vi "Sequence.Compile.vi"(8 "error in (no error)":errorcluster, 11 "State Variables":T10={"Aliases.All"=[], "Aliases.Outputs"=[], "UI.Sequence#ofColumns"=0, "SysDef.Path"=path "", "UI.SequenceRef"=refnum, "UI.StepInformationRef"=refnum, "UI.AbortRef"=refnum, "UI.GraphRef"=refnum, "UI.ViewRef"=refnum, "UI.IterationsRef"=refnum, "UI.IterationInformationRef"=refnum, "INI.Settings"={"Build Location"=path "C:/Simple Sequence Editor/SequenceRepo", "LoggingLocation"=path ""}, "NIVS.Workspace Event"=refnum, "UI.SkipChannel"=refnum, "NIVS.Launched?"=FALSE, "UI.DurationChannel"=refnum}) -> (0 "error out":errorcluster, 1 "Warnings":string[](array[string]), 2 "CompiledSettings":T1)   [LabVIEW 2013, in "Simple Sequence Tools - Editor.lvlib"]
uses:
  Simple Sequence Tools - Editor.lvlib
  Types/Main.StateVariables.ctl
  Shared/Types/Channel.Properties.ctl
  Shared/Types/INI.Settings
  Types/Compiled.RTSequenceProperties.ctl
  Types/Compiled.StepProperties.ctl
  Types/Compiled.IOStateProperties.ctl
  Types/Compiled.StepElementProperties.ctl
  Shared/Types/Step.Types.ctl
  Types/Compiled.StepCondition.ctl
  Types/Conditions.OperationTypes.ctl
  Types/Compiled.SequenceChannels.ctl
  Shared/Simple Sequence Tools - Shared.lvlib
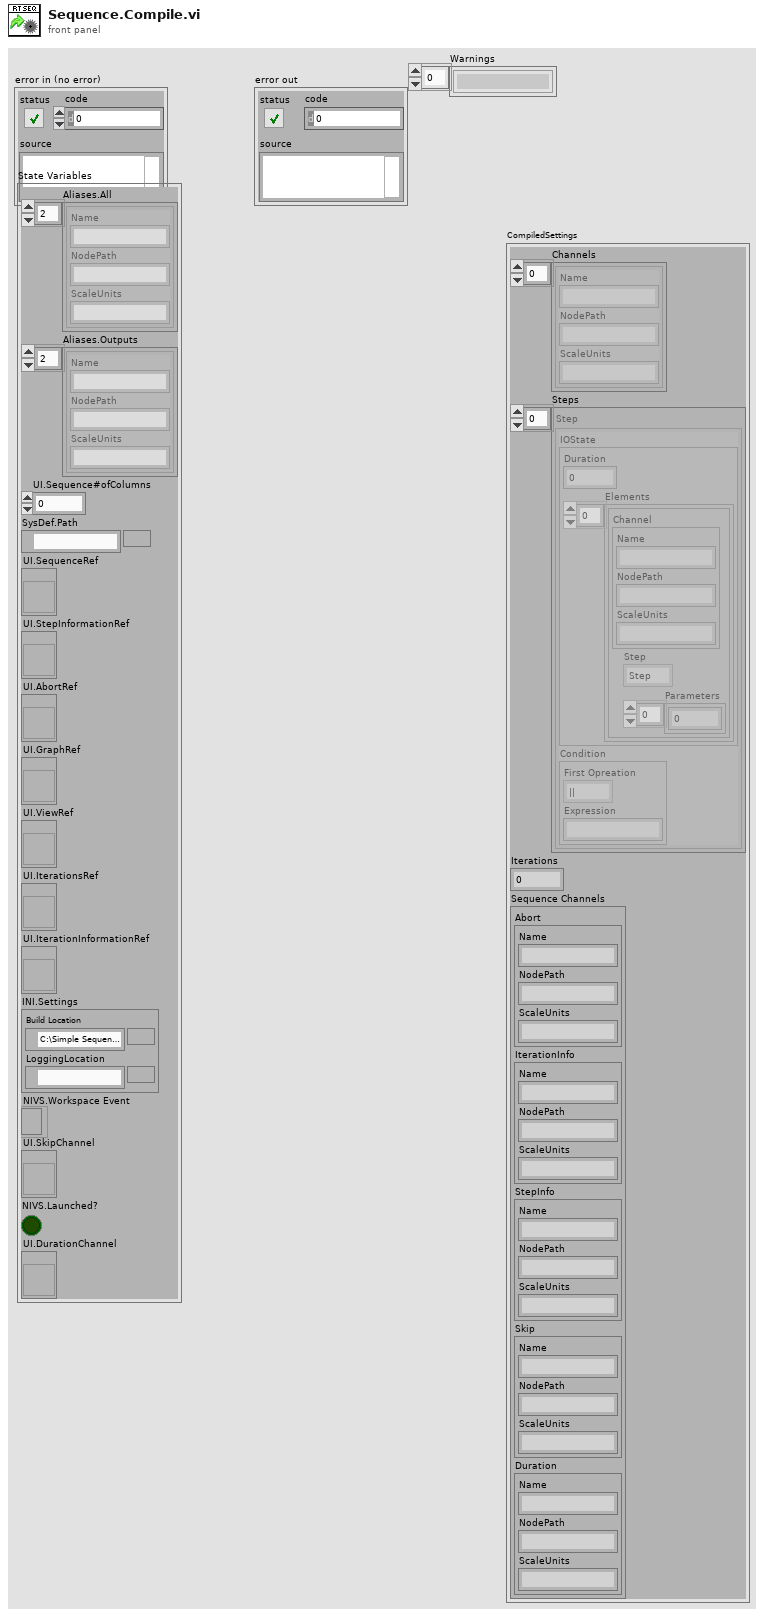
[diagram p1: front panel]
types:
  T1 = typedef "Simple Sequence Tools - Editor.lvlib/Compiled.RTSequenceProperties.ctl" = cluster{"Channels":T2[], "Steps":T3[], "Iterations":u32, "Sequence Channels":T9}
  T2 = typedef "Simple Sequence Tools - Shared.lvlib/Channel.Properties.ctl" = cluster{"Name":string, "NodePath":string, "ScaleUnits":string}
  T3 = typedef "Simple Sequence Tools - Editor.lvlib/Compiled.StepProperties.ctl" = cluster{"IOState":T4, "Condition":T7}
  T4 = typedef "Simple Sequence Tools - Editor.lvlib/Compiled.IOStateProperties.ctl" = cluster{"Duration":dbl, "Elements":T5[]}
  T5 = typedef "Simple Sequence Tools - Editor.lvlib/Compiled.StepElementProperties.ctl" = cluster{"Channel":T2, "Step":T6, "Parameters":dbl[]}
  T6 = typedef "Simple Sequence Tools - Shared.lvlib/Step.Types.ctl" = enum8{"Step", "iStep", "Ramp", "Unchanged", "Unknown", "Sine", "LogSine", "LinearSine", "ForcedRamp"}
  T7 = typedef "Simple Sequence Tools - Editor.lvlib/Compiled.StepCondition.ctl" = cluster{"First Opreation":T8, "Expression":string}
  T8 = typedef "Simple Sequence Tools - Editor.lvlib/Conditions.OperationTypes.ctl" = enum8{"None", "&&", "||"}
  T9 = typedef "Simple Sequence Tools - Editor.lvlib/Compiled.SequenceChannels.ctl" = cluster{"Abort":T2, "IterationInfo":T2, "StepInfo":T2, "Skip":T2, "Duration":T2}
  T10 = typedef "Simple Sequence Tools - Editor.lvlib/Main.StateVariables.ctl" = cluster{"Aliases.All":T2[], "Aliases.Outputs":T2[], "UI.Sequence#ofColumns":i32, "SysDef.Path":path, "UI.SequenceRef":refnum<vi>, "UI.StepInformationRef":refnum<vi>, "UI.AbortRef":refnum<vi>, "UI.GraphRef":refnum<vi>, "UI.ViewRef":refnum<vi>, "UI.IterationsRef":refnum<vi>, "UI.IterationInformationRef":refnum<vi>, "INI.Settings":T11, "NIVS.Workspace Event":refnum<event-registration>, "UI.SkipChannel":refnum<vi>, "NIVS.Launched?":bool, "UI.DurationChannel":refnum<vi>}
  T11 = typedef "Simple Sequence Tools - Shared.lvlib/INI.Settings" = cluster{"Build Location":path, "LoggingLocation":path}
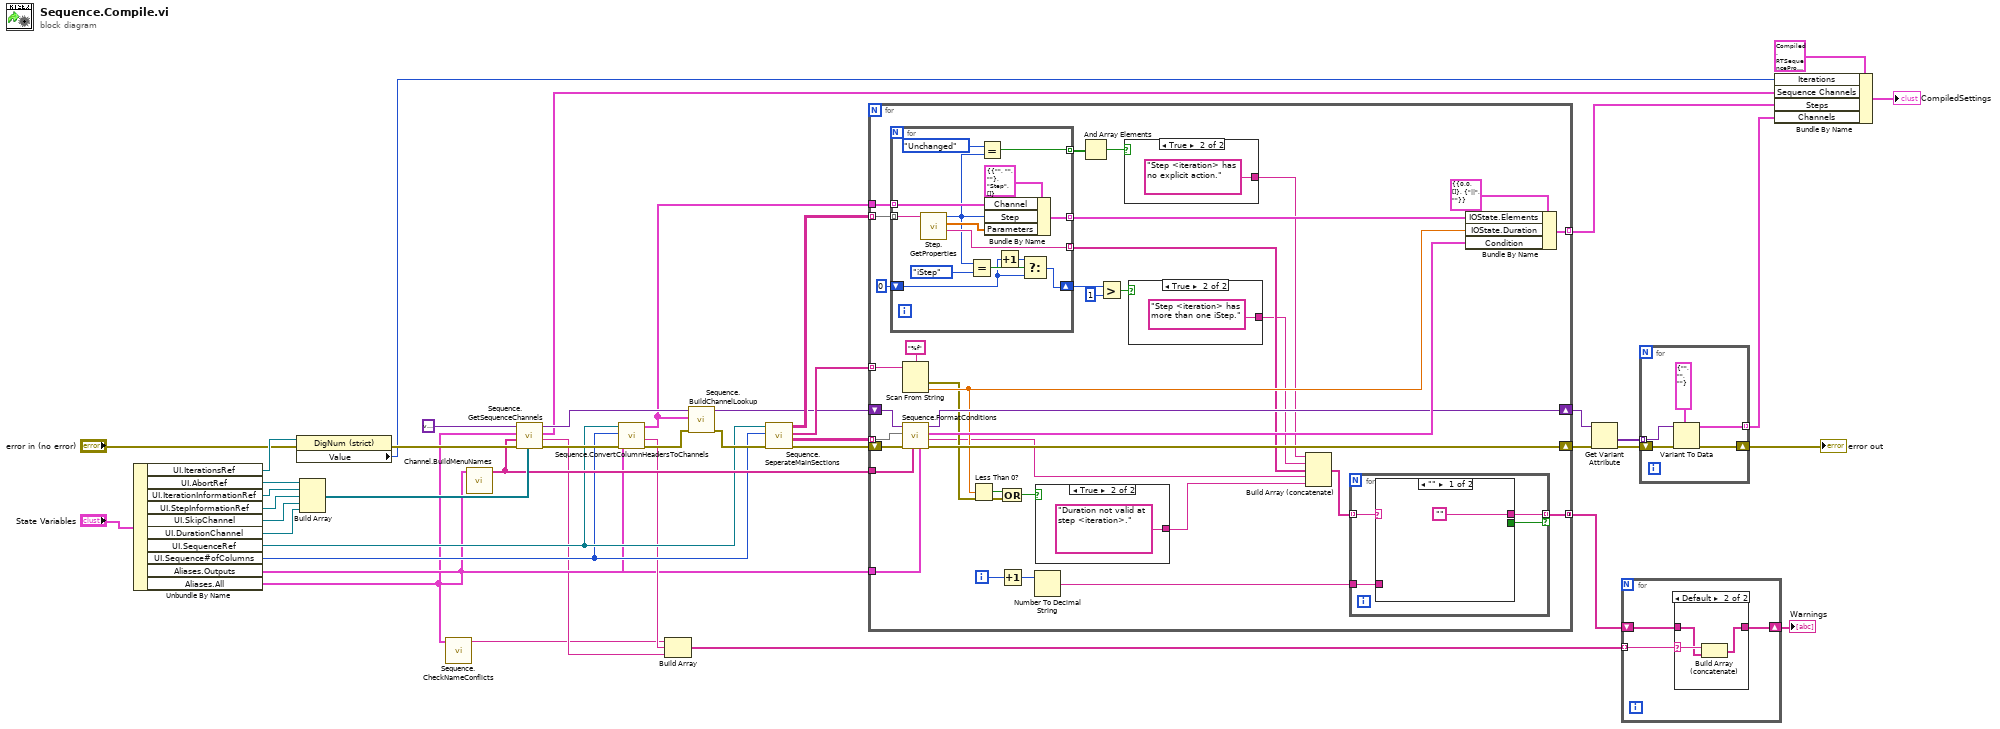
[diagram p0: block diagram]
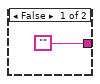
[diagram p3: hidden frame]
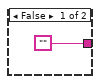
[diagram p4: hidden frame]
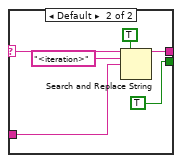
[diagram p5: hidden frame]
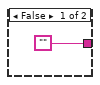
[diagram p6: hidden frame]
diagram:
  n1 = Unbundle By Name("State Variables") -> ("UI.IterationsRef"=w34:refnum<vi>, "UI.AbortRef"=w30:refnum<vi>, "UI.IterationInformationRef"=w29:refnum<vi>, "UI.StepInformationRef"=w28:refnum<vi>, "UI.SkipChannel"=w4:refnum<vi>, "UI.DurationChannel"=w1:refnum<vi>, "UI.SequenceRef"=w12:refnum<vi>, "UI.Sequence#ofColumns"=w11:i32, "Aliases.Outputs"=w10:T2[], "Aliases.All"=w3:T2[])
  n2 = property class="DigNum (strict)"(reference=w34, error in="error in (no error)") -> (error out=w27:errorcluster, "Value"=w16:u32)  [unwired: 1 out]
  n3 = Build Array(w30, w29, w28, w4, w1) -> (w26:refnum<vi>[])
  n4 = call "Sequence.CheckNameConflicts.vi"("Aliases.All"=w3) -> ("Warning"=w2:string)  [unwired: 10 in]
  n5 = call "Channel.BuildMenuNames.vi"("Aliases"=w3) -> ("Aliases Array"=w23:string[])  [unwired: 10 in]
  n6 = call "Sequence.GetSequenceChannels.vi"("Refs"=w26, "error in (no error)"=w27, "Aliases Array"=w23, "Aliases.All"=w3, "ChannelsLookup"=variant ("variant")) -> ("error out"=w14:errorcluster, "Warnings"=w8:string, "SequenceChannels"=w24:T9, "ChannelsLookup"=w25:variant)  [unwired: 3 in]
  n7 = call "Sequence.ConvertColumnHeadersToChannels.vi"("error in (no error)"=w14, "Aliases.Outputs"=w10, "UI.Sequence#ofColumns"=w11, "UI.SequenceRef"=w12) -> ("error out"=w13:errorcluster, "Warning"=w9:string, "Output Channels"=w20:T2[])  [unwired: 5 in]
  n8 = Build Array(w2, w9, w8) -> (w7:string[])
  n9 = call "Sequence.BuildChannelLookup.vi"("error in (no error)"=w13, "Output Channels"=w20, "ChannelLookup"=w25) -> ("error out"=w22:errorcluster, "ChannelLookup"=w19:variant)  [unwired: 7 in]
  n10 = call "Sequence.SeperateMainSections.vi"("error in (no error)"=w22, "UI.Sequence#ofColumns"=w11, "MulticolumnListbox in"=w12) -> ("error out"=w21:errorcluster, "Conditions"=w39:string[][], "Duration"=w43:string[], "Steps"=w42:string[][])  [unwired: 5 in]
  n11 = for {
    tunnel: w43 -> [w78] mode=indexing
    tunnel: w42 -> [w77] mode=indexing
    tunnel: w20 -> [w76]
    tunnel: [w73] -> w18 mode=indexing
    tunnel: w39 -> [w68] mode=indexing
    tunnel: w23 -> [w69]
    tunnel: w3 -> [w70]
    shift-right: [w72] -> w32
    shift-left: w21 -> [w75]
    shift-right: [w65] -> w31
    shift-left: w19 -> [w67]
    tunnel: [w52] -> w6 mode=concatenating
    i -> [w55]
    n12 = for {
      tunnel: w77 -> [w109] mode=indexing
      tunnel: w76 -> [w107] mode=indexing
      tunnel: [w105] -> w71 mode=indexing
      tunnel: [w104] -> w57 mode=indexing
      shift-right: [w101] -> w50
      shift-left: 0 -> [w100]
      tunnel: [w96] -> w46 mode=indexing
      n13 = call "Step.GetProperties.vi"("String in"=w109) -> ("Warning"=w104:string, "Parameters"=w106:dbl[], "Step"=w98:T6)  [unwired: 8 in]
      n14 = Equal?(x=w98, y=Step.Types."iStep") -> (x = y?=w102:bool)
      n15 = Equal?(x=Step.Types."Unchanged", y=w98) -> (x = y?=w96:bool)
      n16 = Bundle By Name(cluster=T5 {"Channel"={"Name"="", "NodePath"="", "ScaleUnits"=""}, "Step"=enum."Step", "Parameters"=[]}, "Channel"=w107, "Step"=w98, "Parameters"=w106) -> (w105:T5)
      n17 = Increment(x=w100) -> (x+1=w99:i32)
      n18 = Select(t=w99, s=w102, f=w100) -> (s? t:f=w101:i32)
    }
    n19 = Scan From String(format string="%f", input string=w78) -> (error out=w61:errorcluster, output 1=w63:dbl)  [unwired: 3 in, 2 out]
    n20 = call "Sequence.FormatConditions.vi"("Aliases.All"=w70, "Aliases Array"=w69, "error in (no error)"=w75, "Conditions"=w68, "variant in"=w67) -> ("error out"=w72:errorcluster, "Warning"=w58:string, "Condition"=w66:T7, "variant out"=w65:variant)  [unwired: 3 in]
    n21 = Less Than 0?(x=w63) -> (x < 0?=w62:bool)
    n22 = Increment(x=w55) -> (x+1=w54:i32)
    n23 = Compound Arithmetic op=OR(w62, w61) -> (w60:bool)
    n24 = Number To Decimal String(number=w54) -> (decimal integer string=w53:string)  [unwired: 1 in]
    n25 = case shown="True" w60 {
      tunnel: ["" "Duration not valid at step <iteration>."] -> w59
      frame False {
      }
      frame True {
      }
    }
    n26 = And Array Elements(Boolean array=w46) -> (logical AND=w45:bool)
    n27 = Greater?(x=w50, y=1) -> (0:w48:bool)
    n28 = case shown="True" w45 {
      tunnel: ["" "Step <iteration> has no explicit action."] -> w44
      frame False {
      }
      frame True {
      }
    }
    n29 = case shown="True" w48 {
      tunnel: ["" "Step <iteration> has more than one iStep."] -> w47
      frame False {
      }
      frame True {
      }
    }
    n30 = Build Array (concatenate)(w44, w47, w57, w58, w59) -> (w56:string[])
    n31 = for {
      tunnel: w56 -> [w85] mode=indexing
      tunnel: w53 -> [w86]
      tunnel: [w84] -> w52 mode=indexing if=w83
      n32 = case shown="\"\"" w85 {
        selector: w85 -> [_ w90]
        tunnel: w86 -> [_ w91]
        tunnel: ["" w89] -> w84
        tunnel: [_ TRUE] -> w83
        frame "" {
        }
        frame Default {
          n33 = Search and Replace String(replace all?=TRUE ("replace all? (F)"), input string=w90, search string="<iteration>", replace string=w91) -> (result string=w89:string)  [unwired: 4 in, 3 out]
        }
      }
    }
    n34 = Bundle By Name(cluster=T3 {"IOState"={"Duration"=0.0, "Elements"=[]}, "Condition"={"First Opreation"=enum."||", "Expression"=""}} ("Step"), "IOState.Elements"=w71, "IOState.Duration"=w63, "Condition"=w66) -> (w73:T3)
  }
  n35 = Get Variant Attribute(Variant=w31, error in=w32) -> (values=w37:variant[], error out=w36:errorcluster)  [unwired: 2 in, 2 out]
  n36 = for {
    tunnel: w7 -> [w112] mode=indexing
    shift-right: [w110] -> w5
    shift-left: w6 -> [w111]
    n37 = case shown="Default" w112 {
      selector: w112 -> [_ w116]
      tunnel: w111 -> [w113 w115]
      tunnel: [w113 w114] -> w110
      frame "" {
      }
      frame Default {
        n38 = Build Array (concatenate)(w116, w115) -> (w114:string[])
      }
    }
  }
  "Warnings" <- w5
  n39 = for {
    tunnel: w37 -> [w121] mode=indexing
    shift-right: [w119] -> w35
    shift-left: w36 -> [w120]
    tunnel: [w117] -> w17 mode=indexing
    n40 = Variant To Data(error in=w120, type=T2 {"Name"="", "NodePath"="", "ScaleUnits"=""} ("cluster"), Variant=w121) -> (data=w117:T2, error out=w119:errorcluster)
  }
  "error out" <- w35
  n41 = Bundle By Name(cluster=T1 {"Channels"=[], "Steps"=[], "Iterations"=0, "Sequence Channels"={"Abort"={"Name"="", "NodePath"="", "ScaleUnits"=""}, "IterationInfo"={"Name"="", "NodePath"="", "ScaleUnits"=""}, "StepInfo"={"Name"="", "NodePath"="", "ScaleUnits"=""}, "Skip"={"Name"="", "NodePath"="", "ScaleUnits"=""}, "Duration"={"Name"="", "NodePath"="", "ScaleUnits"=""}}}, "Iterations"=w16, "Sequence Channels"=w24, "Steps"=w18, "Channels"=w17) -> (→"CompiledSettings":T1)
